vi "北斗初始化变量 (子VI).vi"(8 "错误输入（无错误）":errorcluster) -> (0 "错误输出":errorcluster)   [LabVIEW 2016, in "环境动力监测库.lvlib" / "NMEA.lvlib"]
uses:
  NMEA.lvlib
  <vilib>/Utility/config.llb/NI_LVConfig.lvlib
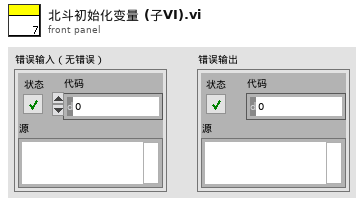
[diagram p1: front panel]
types:
  T1 = cluster{"监测项描述:输出":string, "连接方式":enum16{"串口", "TCP"}, "端口":string, "IP address:":string, "Port:":string, "站号":u64, "传感器型号":string, "波特率":u64, "data bits":u64, "停止位":u16, "奇偶校验":u16, "声光告警启用":bool}
  T2 = typedef "NI_LVConfig.lvlib/Config Data RefNum.ctl" = refnum<k1>
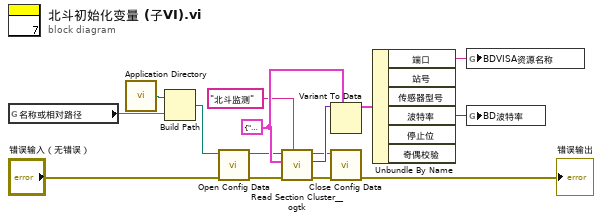
[diagram p0: block diagram]
diagram:
  w11 = T1 {"监测项描述:输出"="", "连接方式"=enum."串口", "端口"="", "IP address:"="", "Port:"="", "站号"=19200, "传感器型号"="", "波特率"=19200, "data bits"=8, "停止位"=10, "奇偶校验"=0, "声光告警启用"=FALSE} ("输入簇")
  n1 = global read "内部交互全局变量.vi" "名称或相对路径"() -> (w1:string)
  n2 = call <vilib>:"Application Directory.vi"() -> ("Application Directory"=w5:path)
  n3 = Build Path(base path=w5, name or relative path=w1) -> (appended path=w4:path)
  n4 = call <vilib>:"Open Config Data.vi"("error in (no error)"="错误输入（无错误）", "configuration file path"=w4) -> ("error out"=w3:errorcluster, "refnum"=w2:T2)  [unwired: 7 in, 1 out]
  n5 = call <userlib>:"Read Section Cluster__ogtk.vi"("section (optional)"="北斗监测", "error in (no error)"=w3, "Section Formatted Cluster Type"=w11, "refnum"=w2) -> ("error out"=w8:errorcluster, "Section Formatted Cluster"=w9:variant, "dup refnum"=w7:T2)  [unwired: 3 in, 2 out]
  n6 = Variant To Data(type=w11, Variant=w9) -> (data=w10:T1)  [unwired: 1 in, 1 out]
  n7 = call <vilib>:"Close Config Data.vi"("error in (no error)"=w8, "refnum"=w7) -> ("error out"=→"错误输出":errorcluster)  [unwired: 8 in, 1 out]
  n8 = Unbundle By Name(w10) -> ("端口"=w12:string, "波特率"=w13:u64)  [unwired: 4 out]
  n9 = global write "断电保存全局变量.vi" "BDVISA资源名称"(w12) -> ()
  n10 = global write "断电保存全局变量.vi" "BD波特率"(w13) -> ()
